vi "Sensors.vi"() -> ()   [LabVIEW 2019]
panel:
  in  "Encoders":T1
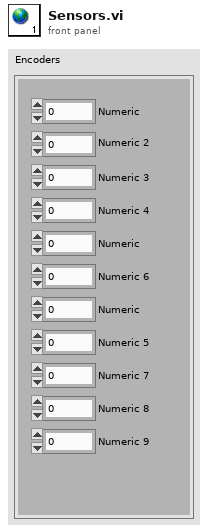
[diagram p1: front panel]
types:
  T1 = cluster{"Numeric":dbl, "Numeric 2":dbl, "Numeric 3":dbl, "Numeric 4":dbl, "Numeric":dbl, "Numeric":dbl, "Numeric 5":dbl, "Numeric 6":dbl, "Numeric 7":dbl, "Numeric 8":dbl, "Numeric 9":dbl}
diagram:
